vi "Parse TXT Configuration File_Read File.vi"(8 "error in (no error)":errorcluster, 11 "file path (use dialog)":path) -> (0 "error out":errorcluster, 3 "Array":string[][](array[string]))   [LabVIEW 2017, in "GE_RM_System Explorer.lvlib"]
uses:
  GE_RM_System Explorer.lvlib
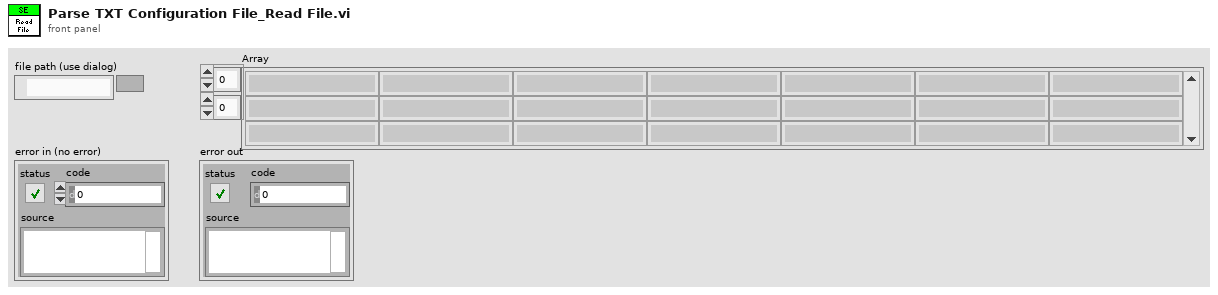
[diagram p1: front panel]
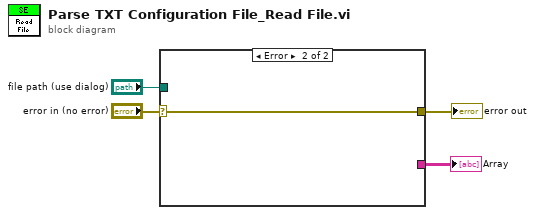
[diagram p0: block diagram]
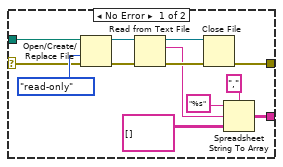
[diagram p2: hidden frame]
diagram:
  n1 = case shown="Error" "error in (no error)" {
    selector: "error in (no error)" -> [w5 w18]
    tunnel: [w17 _] -> w4
    tunnel: [w16 w18] -> w3
    tunnel: "file path (use dialog)" -> [w14 _]
    frame No Error {
      n2 = Open/Create/Replace File(file path (use dialog)=w14, error in=w5, access (0:read/write)=enum16{"read/write", "read-only", "write-only"}."read-only") -> (refnum out=w11:refnum<file>, error out=w12:errorcluster)  [unwired: 3 in, 1 out]
      n3 = Read from Text File(file (use dialog)=w11, error in=w12) -> (refnum out=w10:refnum<file>, text=w7:string, error out=w9:errorcluster)  [unwired: 2 in, 1 out]
      n4 = Close File(refnum=w10, error in=w9) -> (error out=w16:errorcluster)  [unwired: 1 out]
      n5 = Spreadsheet String To Array(delimiter (Tab)=",", format string="%s", spreadsheet string=w7, array type (2D Dbl)=string[][] []) -> (array=w17:string[][])
    }
    frame Error {
    }
  }
  "Array" <- w4
  "error out" <- w3
